vi "New Progress Window.vi"(8 "error in (no error)":errorcluster) -> (0 "error out":errorcluster, 2 "DVRs":T1, 3 "VI refnum":refnum<vi>)   [LabVIEW 2017, in "Build Automation.lvlib"]
uses:
  Build Automation.lvlib
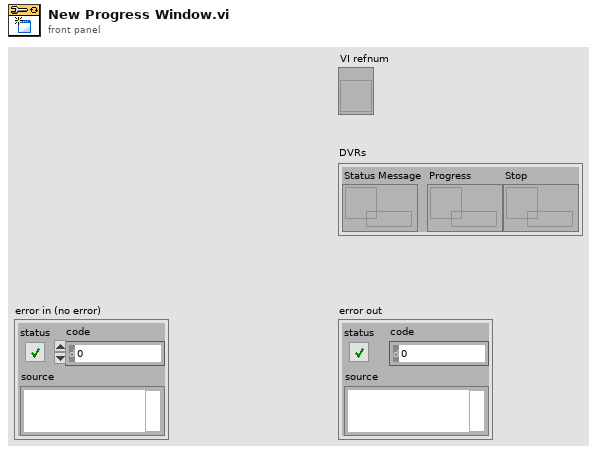
[diagram p1: front panel]
types:
  T1 = cluster{"Status Message":refnum<data-value>, "Progress":refnum<data-value>, "Stop":refnum<data-value>}
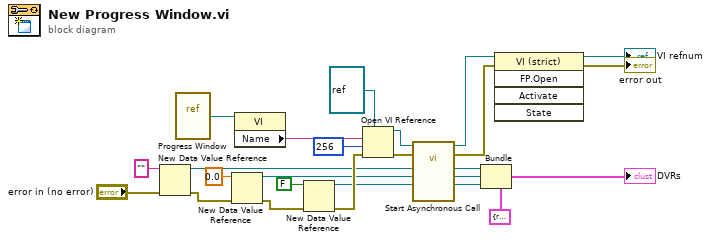
[diagram p0: block diagram]
diagram:
  n1 = New Data Value Reference(data value="", error in="error in (no error)") -> (data value reference=w9:refnum<data-value>, error out=w20:errorcluster)
  n2 = vi-ref "Progress Window.vi"() -> (w2:refnum<vi>)
  n3 = New Data Value Reference(data value=0.0, error in=w20) -> (data value reference=w8:refnum<data-value>, error out=w21:errorcluster)
  n4 = property class="VI"(reference=w2) -> ("Name"=w1:string)  [unwired: 1 in, 2 out]
  n5 = New Data Value Reference(data value=FALSE, error in=w21) -> (data value reference=w10:refnum<data-value>, error out=w13:errorcluster)
  n6 = Open VI Reference(type specifier VI Refnum (for type only)=refnum<vi> refnum, vi path=w1, options=256, error in (no error)=w13) -> (vi reference=w15:refnum<vi>, error out=w16:errorcluster)  [unwired: 2 in]
  n7 = call-by-ref "Start Asynchronous Call"(reference=w15, error in=w16, "Stop"=w10, "Progress"=w8, "Status String"=w9) -> (reference out=w6:refnum<vi>, error out=w4:errorcluster)  [unwired: 9 in]
  n8 = Bundle(cluster=T1 {"Status Message"=refnum, "Progress"=refnum, "Stop"=refnum} ("DVRs"), "Status Message"=w9, "Progress"=w8, "Stop"=w10) -> (→"DVRs":T1)
  n9 = invoke class="VI (strict)" method="FP.Open"(reference=w6, error in=w4) -> (reference out=→"VI refnum":refnum<vi>, error out=→"error out":errorcluster)  [unwired: 3 in, 3 out]
